vi "Comma separated string to string array.vi"(11 "Channel(s)":string) -> (3 "Array":string[](array[string]))   [LabVIEW 2018]
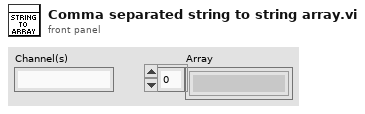
[diagram p1: front panel]
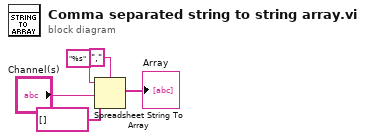
[diagram p0: block diagram]
diagram:
  n1 = Spreadsheet String To Array(delimiter (Tab)=",", format string="%s", spreadsheet string="Channel(s)", array type (2D Dbl)=string[] []) -> (array=→"Array":string[])
